vi "DispenseOn_WaitTime.vi"(8 "error in (no error)":errorcluster, 10 "milliseconds to wait":u32, 11 "I-O in":refnum<class "Copy of I-O.lvclass">) -> (0 "error out":errorcluster, 3 "I-O out":refnum<class "Copy of I-O.lvclass">)   [LabVIEW 2016]
uses:
  Copy of I-O.lvclass
panel:
  # "Dispense On for ... millisecond"
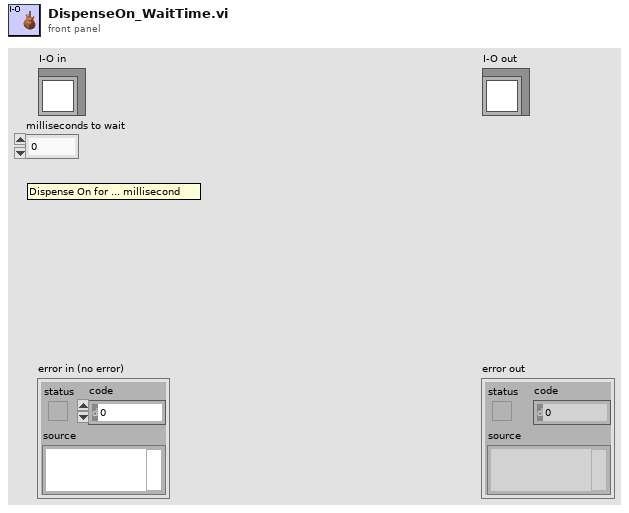
[diagram p1: front panel]
types:
  T1 = typedef "Copy of I-O.lvclass/Pin Map.ctl" = cluster{"Region Valves":i32[], "Extra Valves":dbl[][], "Tool Primary Valve":i32, "Tool Secondary Valve":i32, "Region Sensors":i32[], "Extra Sensors":dbl[][], "Tool Primary Sensor":dbl, "Tool Secondary Sensor":dbl, "Compression Sensor":dbl, "5V":i32, "NTU_Glue":dbl}
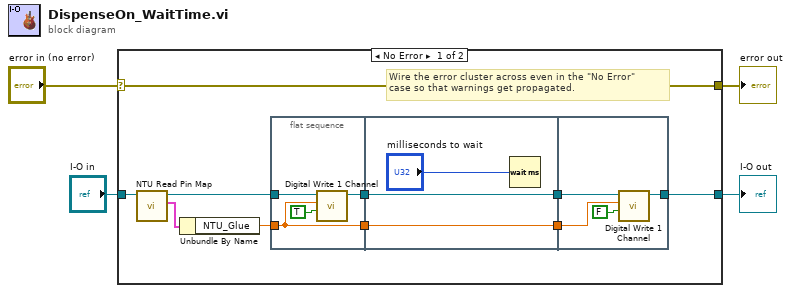
[diagram p0: block diagram]
diagram:
  n1 = case shown="No Error" "error in (no error)" {
    selector: "error in (no error)" -> [w14 w27]
    tunnel: [w14 w27] -> w3
    tunnel: [w12 w26] -> w1
    tunnel: "I-O in" -> [w7 w26]
    frame No Error {
      # "Wire the error cluster across even in the \"No Error\"\ncase so that warnings get propagated."
      n2 = call-dynamic "NTU Read Pin Map.vi"("I-O in"=w7) -> ("Pin Map"=w5:T1, "I-O out"=w6:refnum<class "Copy of I-O.lvclass">)  [unwired: 8 in, 1 out]
      n3 = Unbundle By Name(w5) -> ("NTU_Glue"=w13:dbl)
      n4 = flat-sequence {
        tunnel: w13 -> [w15]
        tunnel: w6 -> [w18]
        tunnel: [w17] -> w11
        tunnel: [w15] -> w9
        tunnel: w11 -> [w21]
        tunnel: [w21] -> w10
        tunnel: w9 -> [w19]
        tunnel: [w19] -> w8
        tunnel: [w24] -> w12
        tunnel: w10 -> [w25]
        tunnel: w8 -> [w23]
        frame #0 {
          n5 = call-dynamic "Digital Write 1 Channel.vi"("Value"=TRUE, "Channel"=w15, "I-O.lvclass"=w18) -> ("I-O.lvclass 2"=w17:refnum<class "Copy of I-O.lvclass">)  [unwired: 7 in, 1 out]
        }
        frame #1 {
          n6 = Wait (ms)(milliseconds to wait="milliseconds to wait") -> ()  [unwired: 1 out]
        }
        frame #2 {
          n7 = call-dynamic "Digital Write 1 Channel.vi"("Value"=FALSE, "Channel"=w23, "I-O.lvclass"=w25) -> ("I-O.lvclass 2"=w24:refnum<class "Copy of I-O.lvclass">)  [unwired: 7 in, 1 out]
        }
      }
    }
    frame Error {
    }
  }
  "error out" <- w3
  "I-O out" <- w1
